vi "Read File+ (string).vi"(5 "convert eol? (no:F)":bool caption="EOL konvertieren? (no:F)", 6 "count":i32 caption="Anzahl", 7 "line mode (characters:F)":bool caption="Zeilenmodus (Zeichen:F)", 8 "error in (no error)":errorcluster caption="Fehler (Eingang, kein Fehler)", 9 "pos offset (bytes:0)":i32 caption="Pos.-Offset (Bytes:0)", 10 "pos mode (rel. to current:2)":enum16{"start", "end", "current"}(ring)=enum."current" caption="Pos.-Modus (relativ zur aktuellen Pos.:2)", 11 "refnum":refnum<file> caption="RefNum") -> (0 "error out":errorcluster caption="Fehler (Ausgang)", 1 "mark after read (bytes)":i32 caption="Dateimarke nach Lesevorgang (Byte)", 2 "string":string caption="String", 3 "dup refnum":refnum<file> caption="RefNum (Kopie)", 4 "EOF?":bool caption="Dateiende?")   [LabVIEW 2009]
doc: "Liest an der angegebenen Stelle einen String aus einer Byte-Stream-Datei; der voreingestellte Platz ist die aktuelle Markierung. Das VI überprüft eingehende und interne Fehler und liest nicht, wenn ein Eingangsfehler auftritt.\n\n'RefNum' ist die Referenz zur geöffneten Datei.\n\n'Pos.-Modus' legt fest, an welcher Stelle, relativ zu 'Pos.-Offset', zu lesen begonnen wird:\n\n 0: am Anfang der Datei plus Pos.-Offest.\n\n 1: am Ende der Datei plus Pos.-Offest.\n\n 2: an der aktuellen Markierung plus Pos.-Offset. Dies ist die Standardeinstellung.\n\nPos.-Offset legt in Byte fest, wie weit entfernt von Pos.-Modus begonnen wird. Der Voreinstellung ist 0.\n\nAnzahl ist die Anzahl der zu lesenden Bytes\n\nZeilenmodus Setze TRUE zu lesen bis eine Zeilenmarke oder ein Zeilenende erreicht ist oder die Zeichenanzahl gelesen wurde. Setze FALSE (Standardwert) zum lesen bis die Zeichenanzahl gelesen wurde oder das Zeilenende erreicht ist. Eine Zeilenmarke ist ein Zeilenumbruch, Zeilenvorschub oder ein Zeilenumbruch gefolgt von einem Zeilenvorschub.\n\nWenn \"EOL umwandeln\" TRUE ist, werden die plattformspezifische Zeilenmarken in LabVIEW-Zeilenmarken konvertiert. Führt bei FALSE (Standardwert) keine Aktion aus.\n\nFehlereingang ist ein Cluster mit 3 Elementen (Fehler?, Code, und Quelle), das den bisherigen Fehlerstatus beschreibt, wenn bei vorher ausgeführten VIs ein Fehler aufgetreten ist. Trat kein Fehler auf, wird das VI normal ausgefürt; Trat ein Fehler auf, wird die Fehlermeldung weitergegeben. Fehler? ist TRUE wenn ein Fehler aufgetreten ist; die Voreinstellung ist FALSE. Code ist der Fehlercode; die Voreinstellung ist 0. Quelle ist in den meisten Fällen der Name des VIs oder der Funktion in der der Fehler aufgetreten ist; die Voreinstellung ist ein leerer String.\n\nRefNum (Kopie) ist ein weitergeleiteter Parameter, der den gleichen Wert wie RefNum hat.\n\nZeichen-String sind die aus der Datei gelesenen Daten.\n\nDateimarke nach Lesevorgang ist die Position der Dateimarke nach dem Lesen. Sie zeigt auf das Zeichen in der Datei, das auf das zuletzt gelesene Zeichen folgt\n\nFehlerausgang ist ein Cluster mit 3 Elementen (Fehler?, Code, und Quelle), das bei der Ausführung des VIs aufgetretene Fehler beschreibt. Wenn kein Eingangsfehler auftrat, wird das VI normal ausgeführt und der Fehlerausgang enthält den Fehlerstatus dieses VIs; wenn ein Eingangsfehler auftrat wird diesen an den Fehlerausgang weitergegeben."
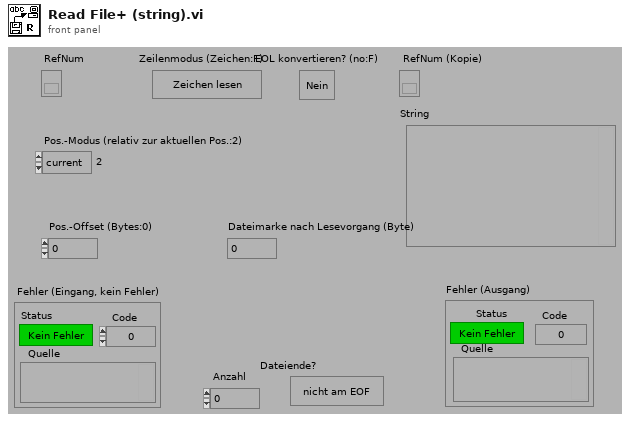
[diagram p1: front panel]
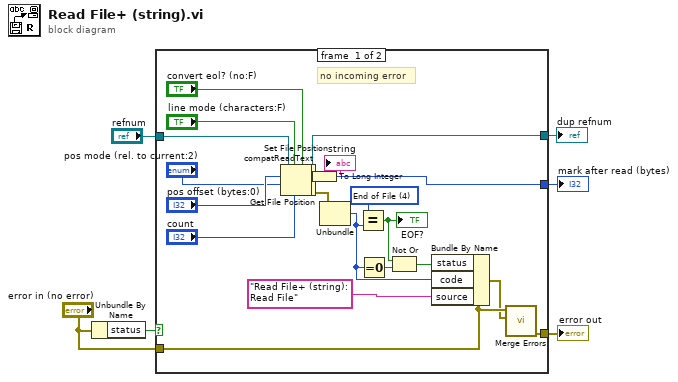
[diagram p0: block diagram]
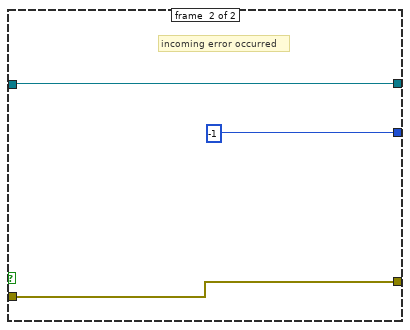
[diagram p2: hidden frame]
diagram:
  n1 = Unbundle By Name("error in (no error)") -> ("status"=w6:bool)
  n2 = case shown="False" w6 {
    tunnel: [w15 w32] -> w5
    tunnel: [w29 -1] -> w4
    tunnel: [w27 w31] -> w3
    tunnel: "refnum" -> [w28 w31]
    tunnel: "error in (no error)" -> [w14 w32]
    frame #0 {
      w20 = 4 items=["No Error", "Manager Argument Error", "Memory Full", "Out of Zone", "End of File", "File Already Open", "Generic File IO Error", "File Not Found", "File Permission Error", "Disk Full", "Duplicate Path", "Too Many Files Open", "Not Enabled", "Resource File Not Found", "Cannot Add Resource", "Resource Not Found", "Image Not Found", "Image Memory Error", "Pen Does Not Exist", "Config Bad Type", "Config Token Not Found", "Config Parse Error", "Config Memory Error", "Bad External Code Format", "Bad External Code Offset", "External Code Not Present", "Null Window", "Destroy Window Mixup", "Null Menu", "Print Aborted", "Bad Print Record", "Print Driver Error", "Windows Error During Print", "Memory Error During Print", "Print Dialog Error", "Generic Print Error", "Invalid Device Refnum", "Device Not Found", "Device Parameter Error", "Device Unit Error", "Can't Open Device", "Device Call Aborted", "Generic Error", "Cancelled By User", "Object ID Too Low", "Object ID Too High", "Object Not In Heap", "Unknown Heap", "Bad DefProc ID", "DefProc Not In Table", "Message Out Of Range", "Null Method", "Unknown Message", "Manager Call Not Supported"]
      # "no incoming error"
      n3 = Set File Position(offset (in bytes) (0)="pos offset (bytes:0)", refnum=w28, from (0:start)="pos mode (rel. to current:2)") -> (refnum out=w11:refnum<file>, error out=w10:errorcluster)  [unwired: 1 in]
      n4 = call <vilib>:"compatReadText.vi"("convert eol (F)"="convert eol? (no:F)", "count"="count", "line mode (F)"="line mode (characters:F)", "error in"=w10, "refnum"=w11) -> ("error out"=w8:errorcluster, "data"=→"string":string, "dup refnum"=w9:refnum<file>)  [unwired: 4 in]
      n5 = Get File Position(4:w8, 7:w9) -> (0:w19:errorcluster, 2:w7:i64, 3:w27:refnum<file>)
      n6 = To Long Integer(number=w7) -> (32bit integer=w29:i32)
      n7 = Unbundle(w19) -> ("code"=w18:i32)  [unwired: 2 out]
      n8 = Equal?(x=w20, y=w18) -> (x = y?=w22:bool)
      "EOF?" <- w22
      n9 = Equal To 0?(x=w18) -> (x = 0?=w21:bool)
      n10 = Not Or(1:w21, 2:w22) -> (0:w16:bool)
      n11 = Bundle By Name(cluster=w14, "status"=w16, "code"=w18, "source"="Read File+ (string): Read File") -> (w13:errorcluster)
      n12 = call <vilib>:"Merge Errors.vi"("error in 2 (no error)"=w13, "error in 1 (no error)"=w14) -> ("error out"=w15:errorcluster)  [unwired: 5 in]
    }
    frame #1 {
      # "incoming error occurred"
    }
  }
  "error out" <- w5
  "mark after read (bytes)" <- w4
  "dup refnum" <- w3
